vi "CalcPodOutputVoltages.vi"(7 "All Pod State Data":T1(array[cluster]), 9 "Default Runtime (s)":dbl=0.1, 11 "Pod Output Vectors":cluster{"Magnitude":dbl, "Direction":dbl}[](array[cluster])) -> (2 "Setpoint Turret Angles":dbl[](array[numeric]), 3 "Motor Outputs":T2(array[cluster]))   [LabVIEW 2014]
uses:
  Variables/Physical data.vi
  Variables/References.vi
  Math/Physics Calculations/SolveMotor_Volts,Torque.vi
  <vilib>/addons/control/pid/pid.llb/PID (DBL Array).vi
  <vilib>/addons/control/pid/NI_PID_pid.lvlib
panel:
  in  "Static torque on turret":dbl=0.1
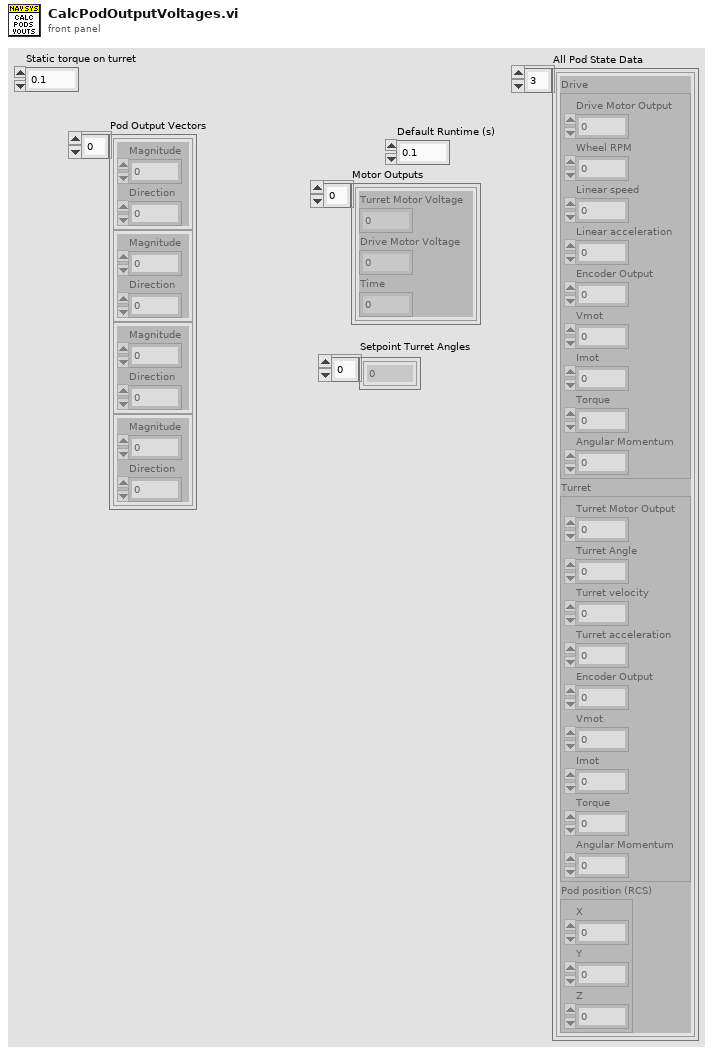
[diagram p1: front panel]
types:
  T1 = cluster{"Drive":cluster{"Drive Motor Output":dbl, "Wheel RPM":dbl, "Linear speed":dbl, "Linear acceleration":dbl, "Encoder Output":dbl, "Vmot":dbl, "Imot":dbl, "Torque":dbl, "Angular Momentum":dbl}, "Turret":cluster{"Turret Motor Output":dbl, "Turret Angle":dbl, "Turret velocity":dbl, "Turret acceleration":dbl, "Encoder Output":dbl, "Vmot":dbl, "Imot":dbl, "Torque":dbl, "Angular Momentum":dbl}, "Pod position (RCS)":cluster{"X":dbl, "Y":dbl, "Z":dbl}}[]
  T2 = cluster{"Turret Motor Voltage":dbl, "Drive Motor Voltage":dbl, "Time":dbl}[]
  T3 = cluster{"PodConfigurations":cluster{"Drive":cluster{"Encoder":cluster{"CPft":dbl, "Location":string, "RIO_PinA":i32, "RIO_PinB":i32, "Invert?":bool}, "Motor":cluster{"PID":cluster{"P":dbl, "I":dbl, "D":dbl}, "CANorPWM Channel":i32, "Invert?":bool, "IsCanSRX?":bool, "Output":cluster{"Max":dbl, "Min":dbl}}}, "Turret":cluster{"Encoder":cluster{"ZeroPosVolts":dbl, "Location":string, "RIO_AnalogChannel":i32, "Invert?":bool}, "Motor":cluster{"PID":cluster{"P":dbl, "I":dbl, "D":dbl}, "CANorPWM Channel":i32, "Invert?":bool, "IsCanSRX?":bool, "Output":cluster{"Max":dbl, "Min":dbl}}}, "Misc":cluster{"Pod_Pos":cluster{"X":dbl, "Y":dbl}, "PDP_Channels":cluster{"Drive":i32, "Turret":i32}}}[], "General Configuration":cluster{"Pod Count":i32, "PDP CAN ID":i32, "PCM CAN ID":i32, "BaseRobotMass":dbl}}
  T4 = cluster{"Drive":cluster{"Encoder":cluster{"CPft":dbl, "Location":string, "RIO_PinA":i32, "RIO_PinB":i32, "Invert?":bool}, "Motor":cluster{"PID":cluster{"P":dbl, "I":dbl, "D":dbl}, "CANorPWM Channel":i32, "Invert?":bool, "IsCanSRX?":bool, "Output":cluster{"Max":dbl, "Min":dbl}}}, "Turret":cluster{"Encoder":cluster{"ZeroPosVolts":dbl, "Location":string, "RIO_AnalogChannel":i32, "Invert?":bool}, "Motor":cluster{"PID":cluster{"P":dbl, "I":dbl, "D":dbl}, "CANorPWM Channel":i32, "Invert?":bool, "IsCanSRX?":bool, "Output":cluster{"Max":dbl, "Min":dbl}}}, "Misc":cluster{"Pod_Pos":cluster{"X":dbl, "Y":dbl}, "PDP_Channels":cluster{"Drive":i32, "Turret":i32}}}[]
  T5 = cluster{"Free Current":dbl, "Stall Current":dbl, "Stall Torque":dbl, "Free Speed":dbl, "Gear Ratio":dbl, "Efficiency":dbl, "Moment":dbl}
  T6 = cluster{"Motor Voltage":dbl, "Motor Torque":dbl, "Motor Current":dbl, "Motor Speed":dbl, "Power Out":dbl, "Power In":dbl, "Motor Efficiency":dbl}
  T7 = cluster{"output":dbl, "Magnitude":dbl, "dt out (s)":dbl}
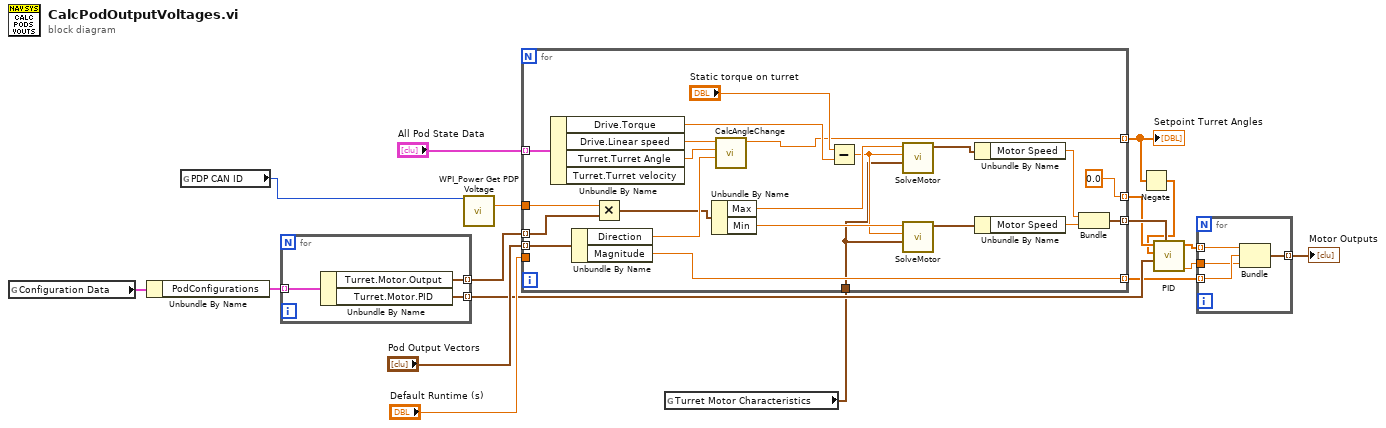
[diagram p0: block diagram]
diagram:
  n1 = global read "Physical data.vi" "Configuration Data"() -> (w17:T3)
  n2 = Unbundle By Name(w17) -> ("PodConfigurations"=w16:T4)
  n3 = global read "References.vi" "PDP CAN ID"() -> (w4:i32)
  n4 = for {
    tunnel: w16 -> [w21] mode=indexing
    tunnel: [w19] -> w10 mode=indexing
    tunnel: [w20] -> w13 mode=indexing
    n5 = Unbundle By Name(w21) -> ("Turret.Motor.Output"=w20:cluster{"Max":dbl, "Min":dbl}, "Turret.Motor.PID"=w19:cluster{"P":dbl, "I":dbl, "D":dbl})
  }
  n6 = call <vilib>:"WPI_Power Get PDP Voltage.vi"("Power Distribution Panel (0)"=w4) -> ("voltage (V)"=w12:dbl)  [unwired: 13 in, 1 out]
  n7 = global read "Physical data.vi" "Turret Motor Characteristics"() -> (w5:T5)
  n8 = for {
    tunnel: "Pod Output Vectors" -> [w42] mode=indexing
    tunnel: "All Pod State Data" -> [w43] mode=indexing
    tunnel: "Default Runtime (s)" -> [_]
    tunnel: [w24] -> w2 mode=indexing
    tunnel: w13 -> [w35] mode=indexing
    tunnel: w12 -> [w36]
    tunnel: [w26] -> w11 mode=indexing
    tunnel: [0.0] -> w3 mode=indexing
    tunnel: [w25] -> w9 mode=indexing
    tunnel: w5 -> [w22]
    n9 = Unbundle By Name(w43) -> ("Drive.Torque"=w38:dbl, "Drive.Linear speed"=w40:dbl, "Turret.Turret Angle"=w39:dbl)  [unwired: 1 out]
    n10 = Unbundle By Name(w42) -> ("Direction"=w41:dbl, "Magnitude"=w25:dbl)
    n11 = Multiply(x=w36, y=w35) -> (x*y=w34:cluster{"Max":dbl, "Min":dbl})
    n12 = Unbundle By Name(w34) -> ("Max"=w33:dbl, "Min"=w32:dbl)
    n13 = call "CalcAngleChange.vi"("Direction"=w41, "Turret Angle"=w39, "Linear speed"=w40) -> ("Angle Change"=w24:dbl)  [unwired: 8 in]
    n14 = Subtract(x="Static torque on turret", y=w38) -> (x-y=w31:dbl)
    n15 = call-poly "SolveMotor.vi"("Motor Characteristics"=w22, "Motor Torque"=w31, "Motor Voltage"=w33) -> ("Motor Data"=w30:T6)  [unwired: 8 in]
    n16 = call-poly "SolveMotor.vi"("Motor Characteristics"=w22, "Motor Torque"=w31, "Motor Voltage"=w32) -> ("Motor Data"=w29:T6)  [unwired: 8 in]
    n17 = Unbundle By Name(w30) -> ("Motor Speed"=w27:dbl)
    n18 = Unbundle By Name(w29) -> ("Motor Speed"=w28:dbl)
    n19 = Bundle("Motor Speed"=w27, "Motor Speed"=w28) -> (w26:cluster{"Motor Speed":dbl, "Motor Speed":dbl})  [unwired: 1 in]
  }
  "Setpoint Turret Angles" <- w2
  n20 = Negate(x=w2) -> (-x=w1:dbl[])
  n21 = call-poly <vilib>:"PID.vi"("output range"=w11, "PID gains"=w10, "process variable"=w1, "setpoint"=w3) -> ("dt out (s)"=w8:dbl, "output"=w7:dbl[])  [unwired: 6 in]
  n22 = for {
    tunnel: w9 -> [w46] mode=indexing
    tunnel: w8 -> [w45]
    tunnel: w7 -> [w47] mode=indexing
    tunnel: [w44] -> w6 mode=indexing
    n23 = Bundle("output"=w47, "Magnitude"=w46, "dt out (s)"=w45) -> (w44:T7)  [unwired: 1 in]
  }
  "Motor Outputs" <- w6
